vi "Load Symbol.vi"(10 "Symbol Folder Path":path, 11 "Tree in":refnum<class "Tree.lvclass">) -> (3 "Tree out":refnum<class "Tree.lvclass">)   [LabVIEW 2024, in "Tree.lvclass"]
uses:
  Tree.lvclass
  Tree.lvclass/Tree.ctl
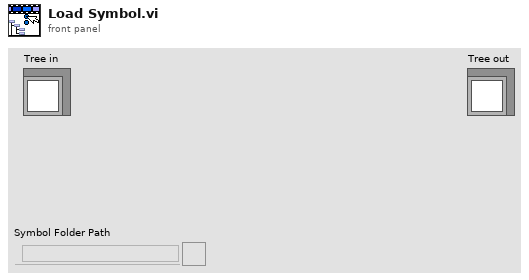
[diagram p1: front panel]
types:
  T1 = typedef "imagedata.ctl" = cluster{"image type":i32, "image depth":i32, "image":u8[], "mask":u8[], "colors":u32[], "Rectangle":cluster{"left":i16, "top":i16, "right":i16, "bottom":i16}}
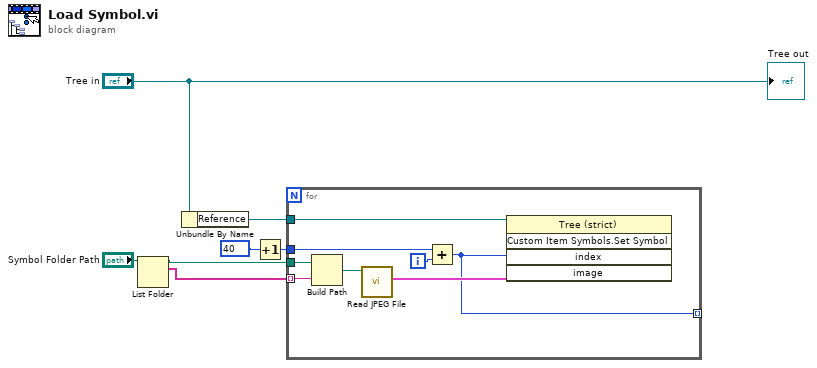
[diagram p0: block diagram]
diagram:
  n1 = List Folder(path="Symbol Folder Path") -> (path out=w4:path, filenames=w3:string[])  [unwired: 3 in, 2 out]
  n2 = Unbundle By Name("Tree in") -> ("Reference"=w6:refnum<vi>)
  n3 = Increment(x=40) -> (x+1=w1:i32)
  n4 = for {
    tunnel: w4 -> [w15]
    tunnel: w3 -> [w12] mode=indexing
    tunnel: w6 -> [w10]
    tunnel: [w9] -> _ mode=indexing
    tunnel: w1 -> [w8]
    i -> [w11]
    n5 = Build Path(base path=w15, name or relative path=w12) -> (appended path=w14:path)
    n6 = call <vilib>:"Read JPEG File.vi"("path to JPEG file"=w14) -> ("image data"=w13:T1)  [unwired: 8 in, 2 out]
    n7 = Add(x=w8, y=w11) -> (x+y=w9:i32)
    n8 = invoke class="Tree (strict)" method="Custom Item Symbols.Set Symbol"(reference=w10, "index"=w9, "image"=w13) -> ()  [unwired: 2 in, 5 out]
  }
  "Tree out" <- "Tree in"
